vi "Init Msg Self.vi"(6 "Actor Msgs":refnum<class "Msg.lvclass">[](array[class]), 9 "Post-Setup Msgs":refnum<class "Msg.lvclass">[](array[class]), 10 "Pre-Setup Msgs":refnum<class "Msg.lvclass">[](array[class])) -> (2 "Msg Self":refnum<class "Msg Self.lvclass">)   [LabVIEW 2020, in "jettl.lvlib" / "Base Msg Self.lvlib"]
uses:
  Base Msg Self.lvlib
  Msg Self/Msg Self.lvclass
  Msg/Msg.lvclass
  Base Msg Self/Base Msg Self.lvclass
  C:/git/jettl/src/jettl/jettl/Msg Self/Msg Self.lvclass
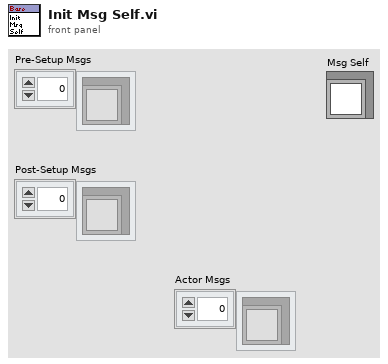
[diagram p1: front panel]
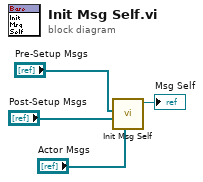
[diagram p0: block diagram]
diagram:
  n1 = call "Init Msg Self.vi"("Actor Msgs"="Actor Msgs", "Post-Setup Msgs"="Post-Setup Msgs", "Pre-Setup Msgs"="Pre-Setup Msgs") -> ("Base Msg Self out"=→"Msg Self":refnum<class "Base Msg Self.lvclass">)  [unwired: 8 in]
